vi "COMI Write8402.vi"(7 "data":i32, 9 "addr":i32, 10 "ch":i32, 11 "hDevice":u32) -> (3 "hDevice out":u32)   [LabVIEW 2017, in "Comidll.lvlib"]
doc: "void (COMI_Write8402) (HANDLE hDevice, int ch, int addr, int data);"
uses:
  <userlib>/Comidll/Comidll.lvlib
  <userlib>/Comidll/Comidll.dll
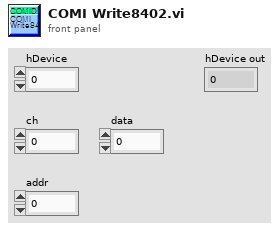
[diagram p1: front panel]
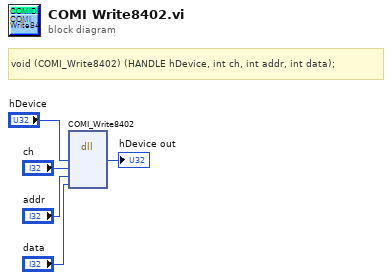
[diagram p0: block diagram]
diagram:
  # "void\t(COMI_Write8402) (HANDLE hDevice, int ch, int addr, int data);"
  n1 = dll-call lib="C:/Program Files/National Instruments/LabVIEW 2017/user.lib/Comidll/Comidll.*" fn="COMI_Write8402"("hDevice"="hDevice", "ch"="ch", "addr"="addr", "data"="data") -> ("hDevice"=→"hDevice out":u32)  [unwired: 7 in, 2 out]
